vi "timedAcq.vi"(8 "error in (no error)":errorcluster, 10 "Time Controls":T1, 11 "SR430Class in":refnum<class "SR430Class.lvclass">) -> (0 "error out":errorcluster, 3 "SR430Class out":refnum<class "SR430Class.lvclass">)   [LabVIEW 2015, in "SR430Class.lvclass"]
uses:
  class/SR430Class.lvclass
  class/SR430Class.lvclass/SR430Class.ctl
  <vilib>/Platform/TimedLoop/XDataNode/timing_clust.ctl
  <vilib>/Platform/TimedLoop/XDataNode/nitl_modes.ctl
  <vilib>/Platform/TimedLoop/XDataNode/wakeup.ctl
  <vilib>/Platform/TimedLoop/scheduler/LVUserAPI/_suppVIs/Create_1kHz_TSource.vi
  <vilib>/express/express arith-compare/Formula/XNode/ExpressFormulaBlockNode.xnode
  <vilib>/platform/TimedLoop/XDataNode/XDataNode.xnode
  support/SR430 Driver/SR430Driver.lvlib
  <vilib>/Platform/TimedLoop/XDataNode/XDNodeRunTimeDep.lvlib
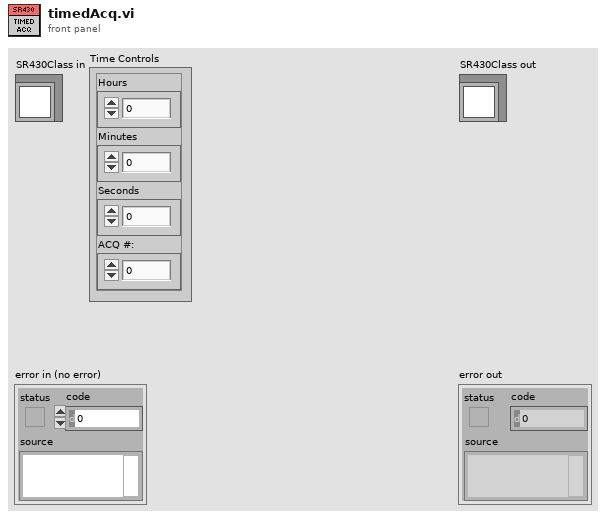
[diagram p1: front panel]
types:
  T1 = cluster{"Hours":dbl, "Minutes":dbl, "Seconds":dbl, "ACQ #:":i32}
  T2 = typedef "XDNodeRunTimeDep.lvlib/timing_clust.ctl" = cluster{"Expected End [f-1]":u64, "Actual End [f-1]":u64, "Finished Late? [f-1]":bool, "Expected End [i-1]":u64, "Actual End [i-1]":u64, "Finished Late? [i-1]":bool, "Expected Start [i]":u64, "Actual Start [i]":u64, "Expected Start [f]":u64, "Actual Start [f]":u64, "Source Name":string, "Structure Name":string, "Period":i64, "Deadline":i64, "Offset":i64, "Start":i64, "Priority":i32, "Timeout":i32, "Mode":T3, "Wakeup Reason":T4, "Error":errorcluster, "Source Type":string, "Secondary Source Type":string, "Global End Time":u64, "Global Start Time":u64, "Frame Duration":u64, "Iteration Duration":u64, "Assigned CPU":i32, "I/O Scan Engine Mode":u32}
  T3 = typedef "XDNodeRunTimeDep.lvlib/nitl_modes.ctl" = enum32{"No Change", "Process missed periods, maintain original phase", "Discard missed periods, maintain original phase", "Process missed periods, ignore original phase", "Discard missed periods, ignore original phase"}
  T4 = typedef "XDNodeRunTimeDep.lvlib/wakeup.ctl" = enum32{"Normal", "Aborted", "Asynchronous wakeup", "Timing source error", "Timed loop error", "Timeout"}
  T5 = typedef "SR430Driver.lvlib/SR430_VISA Control.ctl" = cluster{"VISA resource name":refnum<visa-resource-name>}
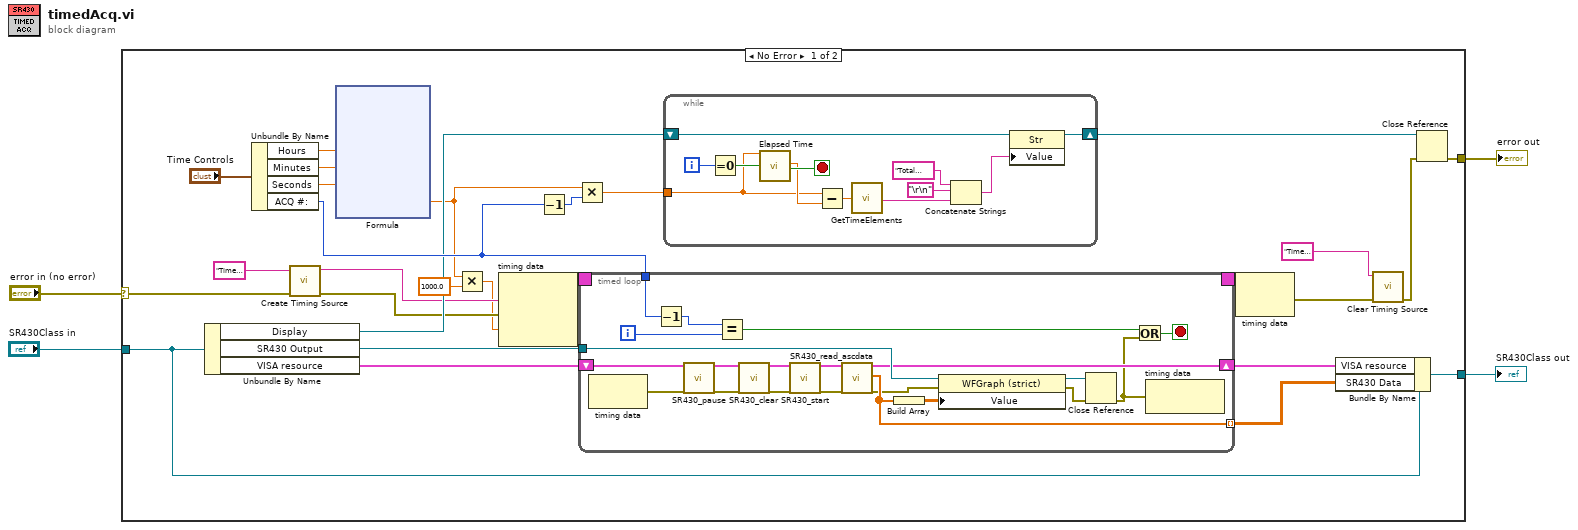
[diagram p0: block diagram]
diagram:
  n1 = case shown="No Error" "error in (no error)" {
    selector: "error in (no error)" -> [w16 w91]
    tunnel: [w18 w91] -> w3
    tunnel: [w28 w90] -> w1
    tunnel: "SR430Class in" -> [w30 w90]
    frame No Error {
      n2 = Unbundle By Name(w30) -> ("Display"=w20:refnum<vi>, "SR430 Output"=w31:refnum<vi>, "VISA resource"=w32:T5)
      n3 = Unbundle By Name("Time Controls") -> ("Hours"=w26:dbl, "Minutes"=w25:dbl, "Seconds"=w24:dbl, "ACQ #:"=w22:i32)
      n4 = call-poly <vilib>:"Create Timing Source.vi"("error in (no error)"=w16, "name (in)"="Timed Acquistion" ("Source Name")) -> ("error out"=w8:errorcluster, "name (out)"=w9:string)  [unwired: 8 in]
      n5 = xnode "Formula"("Hours"=w26, "Min"=w25, "Sec"=w24) -> ("Result"=w15:dbl)  [unwired: 1 in, 1 out]
      n6 = Multiply(x=w15, y=1000.0) -> (x*y=w5:dbl)
      n7 = node-c288(w9, w8, w5) -> (w11:T2)
      n8 = Decrement(x=w22) -> (x-1=w21:i32)
      n9 = Multiply(x=w15, y=w21) -> (x*y=w23:dbl)
      n10 = timed-loop {
        timing: w11 -> [_]
        timing-out: [_] -> w10
        tunnel: w31 -> [w52]
        tunnel: [w50] -> w6 mode=indexing
        tunnel: w22 -> [w49]
        shift-right: [w51] -> w29
        shift-left: w32 -> [w53]
        i -> [w36]
        stop <- w33 stop-if-true
        n11 = node-c288() -> (w35:errorcluster)  [unwired: 1 in]
        n12 = Decrement(x=w49) -> (x-1=w43:i32)
        n13 = call "SR430_pause.vi"("address"=w53, "error in (no error)"=w35) -> ("address out"=w38:T5, "error out"=w37:errorcluster)  [unwired: 16 in]
        n14 = Equal?(x=w43, y=w36) -> (x = y?=w39:bool)
        n15 = call "SR430_clear.vi"("address"=w38, "error in (no error)"=w37) -> ("address out"=w47:T5, "error out"=w48:errorcluster)  [unwired: 16 in]
        n16 = call "SR430_start.vi"("address"=w47, "error in (no error)"=w48) -> ("address out"=w46:T5, "error out"=w45:errorcluster)  [unwired: 16 in]
        n17 = call "SR430_read_ascdata.vi"("address"=w46, "error in (no error)"=w45) -> ("address out"=w51:T5, "Data"=w50:dbl[], "error out"=w44:errorcluster)  [unwired: 14 in, 1 out]
        n18 = Build Array(w50) -> (w40:dbl[][])
        n19 = property class="WFGraph (strict)"(reference=w52, error in=w44, "Value"=w40) -> (reference out=w42:refnum<vi>, error out=w41:errorcluster)
        n20 = Close Reference(reference=w42, error in (no error)=w41) -> (error out=w34:errorcluster)
        n21 = Or(x=w39, y=w34) -> (x .or. y?=w33:bool)
        n22 = node-c288(w34) -> ()  [unwired: 1 out]
      }
      n23 = while {
        tunnel: w23 -> [w70]
        shift-right: [w71] -> w19
        shift-left: w20 -> [w72]
        i -> [w74]
        stop <- w77 stop-if-true
        n24 = Equal To 0?(x=w74) -> (x = 0?=w73:bool)
        n25 = call "Elapsed Time"("Time Target (s)"=w70, "Reset"=w73) -> ("Elapsed Time (s)"=w76:dbl, "Time has Elapsed"=w77:bool)  [unwired: 10 in, 6 out]
        n26 = Subtract(x=w70, y=w76) -> (x-y=w75:dbl)
        n27 = call "GetTimeElements.vi"("SECONDS"=w75) -> ("String (relative time format)"=w66:string)
        n28 = Concatenate Strings("Total Time Remaining:" ("string"), "\r\n", w66) -> (w67:string)
        n29 = property class="Str"(reference=w72, "Value"=w67) -> (reference out=w71:refnum<vi>)  [unwired: 1 in, 1 out]
      }
      n30 = node-c288(w10) -> (w7:errorcluster)
      n31 = Bundle By Name(cluster=w30, "VISA resource"=w29, "SR430 Data"=w6) -> (w28:refnum<class "SR430Class.lvclass">)
      n32 = call <vilib>:"Clear Timing Source.vi"("error in (no error)"=w7, "name"="Timed Acquistion" ("Source Name")) -> ("error out"=w13:errorcluster)  [unwired: 8 in, 1 out]
      n33 = Close Reference(reference=w19, error in (no error)=w13) -> (error out=w18:errorcluster)
    }
    frame Error {
    }
  }
  "error out" <- w3
  "SR430Class out" <- w1
